vi "uTTA_Calibration_V2.vi"() -> ()   [LabVIEW 2021]
uses:
  <vilib>/Utility/miscctls.llb/LVPointTypeDef.ctl
  uTTA_Device_Driver/uTTA_Controls/CTL_uTTA_AnalogParameter.ctl
  uTTA_Device_Driver/uTTA_Controls/CTL_uTTA_OperatingMode.ctl
panel:
  in  "Tab Control":enum32{"Setup", "Calibration"}(tab)
  in  "Embedd Steps":bool caption="Embedd Calibration Steps in Main Window"
  in  "ADC Stage":bool=TRUE
  in  "Heating Current":bool=TRUE
  in  "Differential Amp":bool=TRUE
  in  "I_Sense":bool=TRUE
  in  "VISA DMM":refnum<visa-resource-name>="COM9"
  in  "Storage_Path":path=path "C:/temp/Eigenentwicklungen/GitHub/uTTA/060_Example_Measurement_Data/Calibration"
  in  "VISA Function Gen":refnum<visa-resource-name>="TCPIP0::192.168.1.54::inst0::INSTR"
  in  "uTTA COM":refnum<visa-resource-name>="COM35"
  in  "Start":bool
  out "PGA":i32
  out "Measurement Active":bool
  out "Queue":i32
  out "Communication Error":errorcluster
  out "RunTime Error":errorcluster
  out "Last Message":string
  out "Status":string="Exit"
  in  "stop":bool
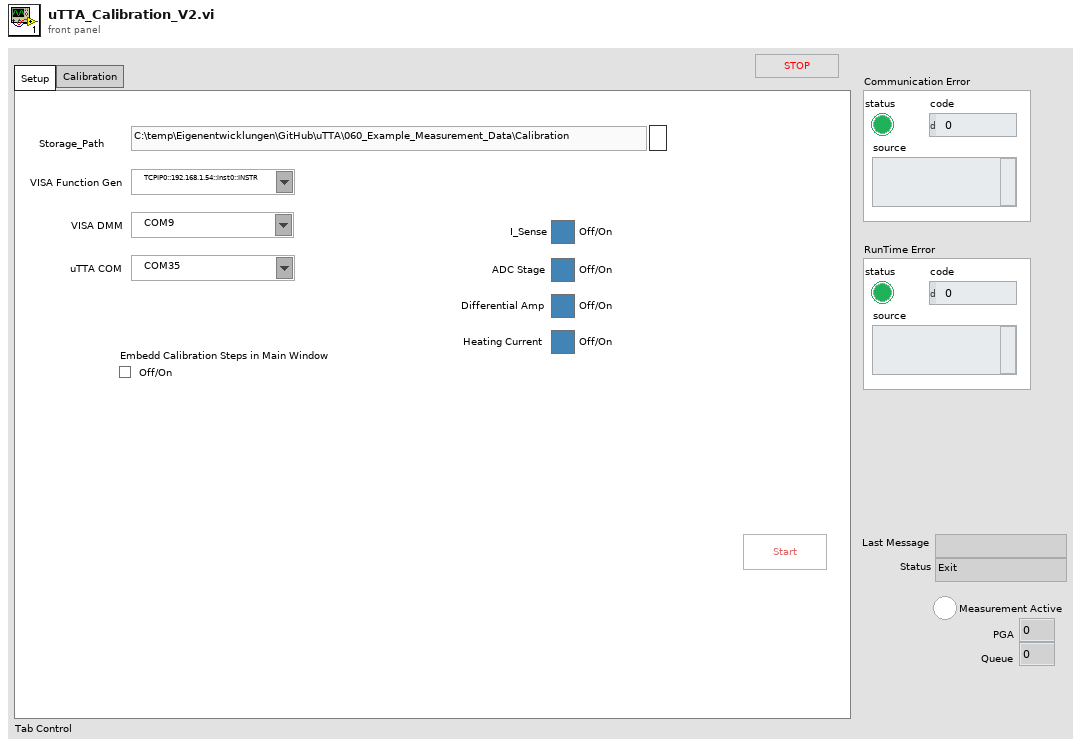
[diagram p1: front panel]
types:
  T1 = typedef "LVPointTypeDef.ctl" = cluster{"Horizontal":i16, "Vertical":i16}
  T2 = cluster{"ADC Values":i16[][], "Temperatures":dbl[][]}
  T3 = enum8{"Enabled", "Disabled", "Disabled and Grayed Out"}
  T4 = enum16{"open", "open or create", "create or replace", "create", "open (read-only)"}
  T5 = typedef "CTL_uTTA_AnalogParameter.ctl" = enum16{"ISEN", "SPARE", "VOFF"}
  T6 = typedef "CTL_uTTA_OperatingMode.ctl" = enum16{"NORMAL", "TEST_MODE", "TEMP_CONTROL"}
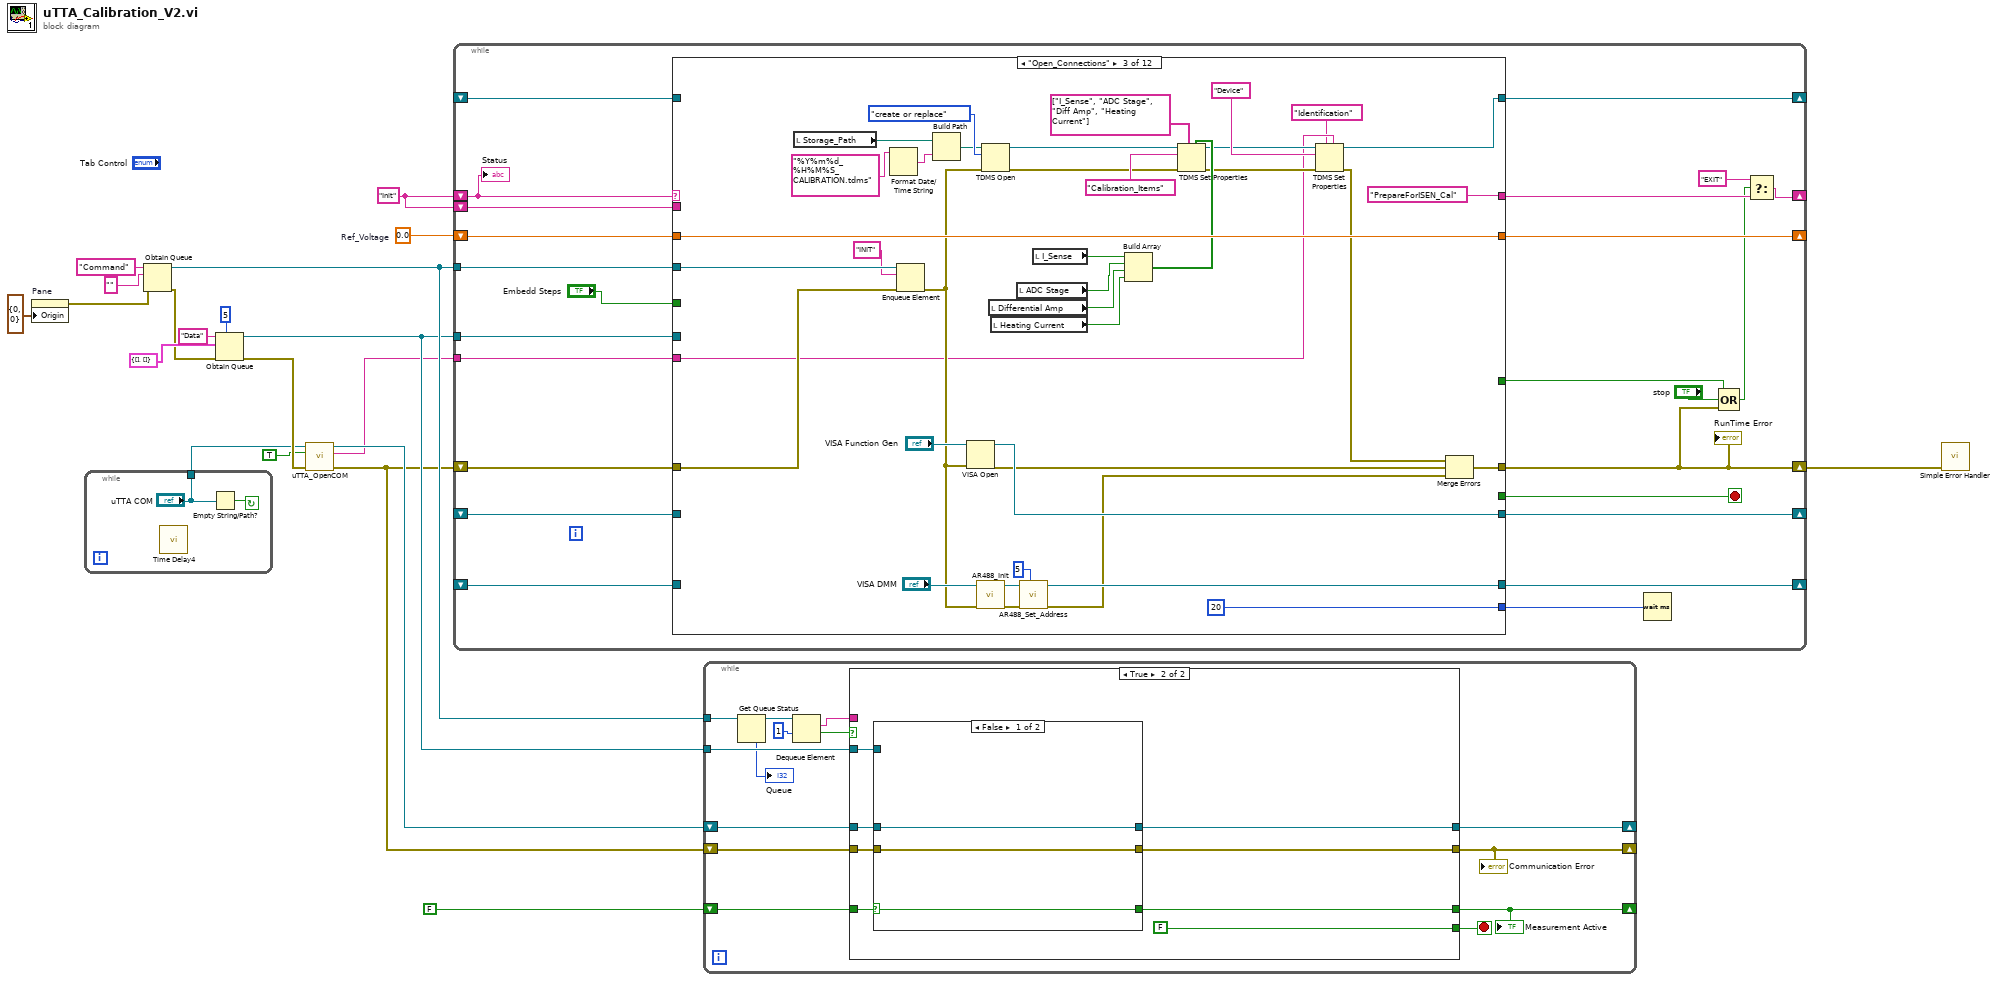
[diagram p0: block diagram]
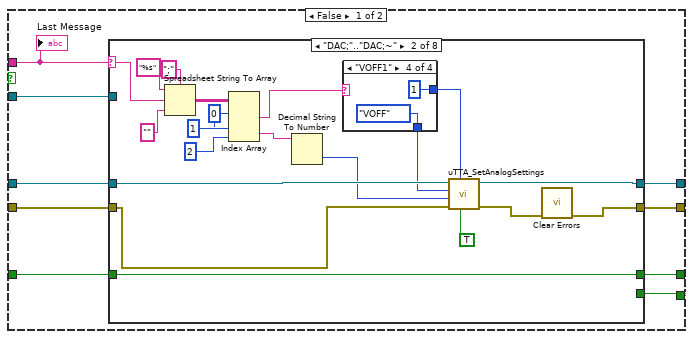
[diagram p2: hidden frame]
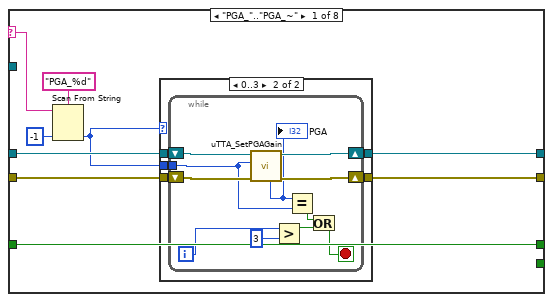
[diagram p3: hidden frame]
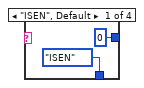
[diagram p5: hidden frame]
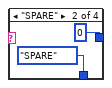
[diagram p6: hidden frame]
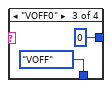
[diagram p7: hidden frame]
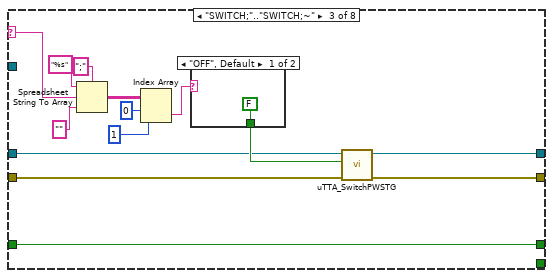
[diagram p8: hidden frame]
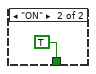
[diagram p9: hidden frame]
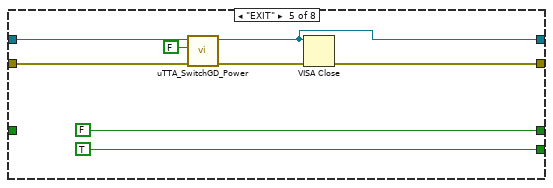
[diagram p11: hidden frame]
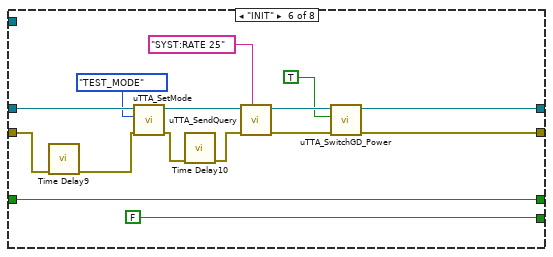
[diagram p12: hidden frame]
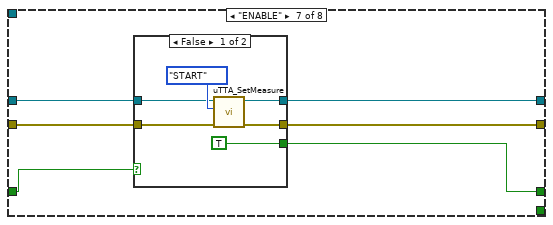
[diagram p13: hidden frame]
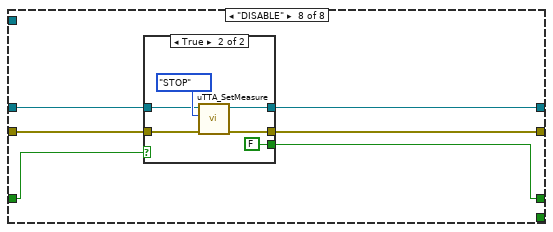
[diagram p15: hidden frame]
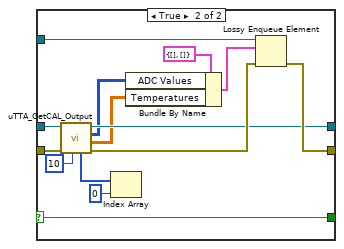
[diagram p17: hidden frame]
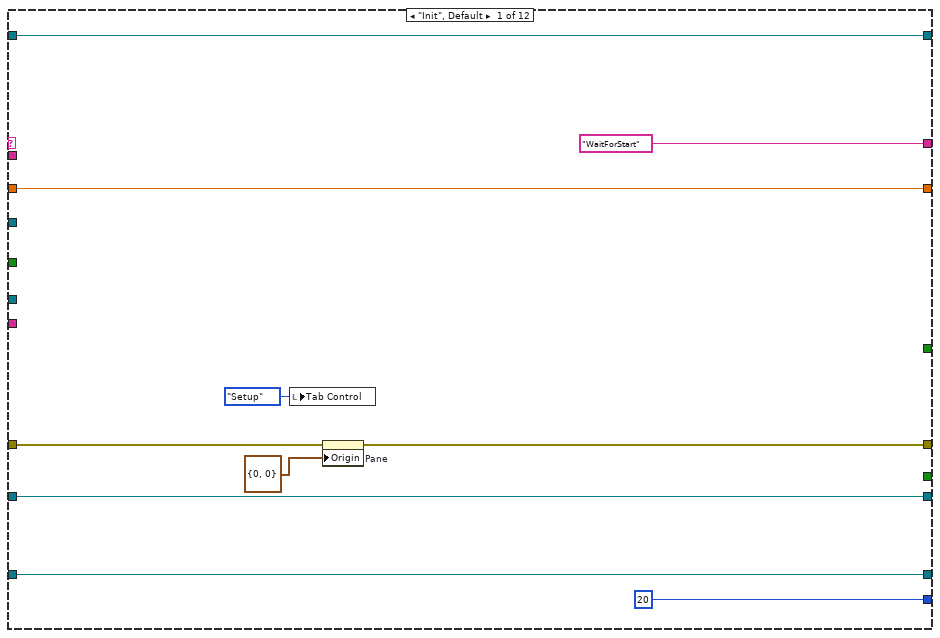
[diagram p18: hidden frame]
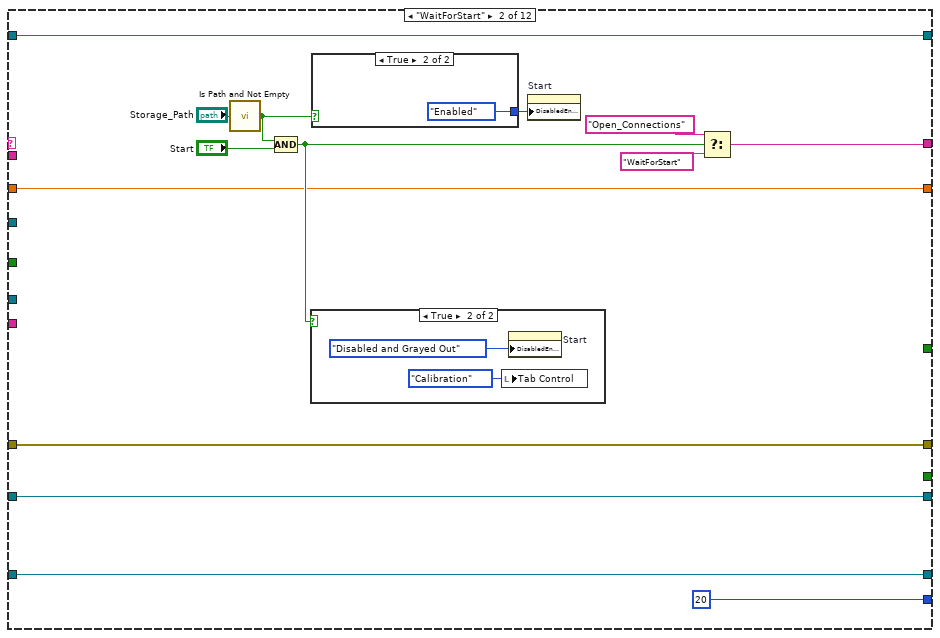
[diagram p19: hidden frame]
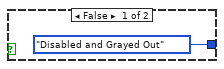
[diagram p20: hidden frame]
diagram:
  w11 = 0.0  # Ref_Voltage
  w10 = "Init"
  n1 = property on="Pane" class="Pane"("Origin"=T1 {"Horizontal"=0, "Vertical"=0}) -> (error out=w4:errorcluster)  [unwired: 2 in, 1 out]
  n2 = while {
    tunnel: ["uTTA COM"] -> w3
    stop <- w22 continue-if-true
    n3 = call "Time Delay4"() -> ()  [unwired: 11 in, 1 out]
    n4 = Empty String/Path?(string/path="uTTA COM") -> (empty?=w22:bool)
  }
  n5 = Obtain Queue(name (unnamed)="Command", element data type="" ("name (unnamed)"), error in (no error)=w4) -> (queue out=w14:refnum<queue>, error out=w15:errorcluster)  [unwired: 2 in, 1 out]
  n6 = Obtain Queue(max queue size (-1, unlimited)=5, name (unnamed)="Data", element data type=T2 {"ADC Values"=[], "Temperatures"=[]}, error in (no error)=w15) -> (queue out=w7:refnum<queue>, error out=w9:errorcluster)  [unwired: 1 in, 1 out]
  n7 = call "uTTA_OpenCOM.vi"("error in"=w9, "Log Serial Monitor(T)"=TRUE ("Log Serial Monitor"), "VISA in"=w3) -> ("error out"=w6:errorcluster, "Identity"=w1:string, "VISA out"=w8:refnum<visa-resource-name>)  [unwired: 6 in]
  n8 = while {
    shift-right: [w33] -> _
    shift-left: w10 -> [w44]
    shift-right: [w31] -> w13
    shift-left: w6 -> [w46]
    shift-right: [w42] -> _
    shift-left: _ -> [w43]
    shift-right: [w41] -> _
    shift-left: _ -> [w40]
    shift-left: w10 -> [w39]
    tunnel: w14 -> [w38]
    tunnel: w7 -> [w37]
    shift-right: [w35] -> _
    shift-left: w11 -> [w36]
    shift-right: [w27] -> _
    shift-left: _ -> [w26]
    tunnel: w1 -> [w23]
    stop <- w28 stop-if-true
    n9 = case shown="\"Open_Connections\"" w44 {
      selector: w44 -> [_ _ _ _ _ _ _ _ _ _ _ w261]
      tunnel: [_ _ _ _ _ _ _ _ _ _ _ TRUE] -> w28
      tunnel: w46 -> [w53 w70 w106 w117 w125 w151 w157 w184 w190 w220 w222 w244]
      tunnel: ["WaitForStart" ("t") w63 "PrepareForISEN_Cal" ("t") w114 "PrepareForADC_Cal" ("t") w147 "PrepareForDiffAmp_Cal" ("t") w180 "Prepare_for_Current_Cal" ("t") w214 "Exit" ("t") w261] -> w34
      tunnel: [w49 w70 w111 w117 w126 w151 w159 w184 w192 w220 w223 w252] -> w31
      tunnel: [u32 20 u32 20 u32 20 u32 20 u32 20 u32 20 u32 20 u32 20 u32 20 u32 10 u32 20 u32 10] -> w45
      tunnel: w43 -> [w52 w62 _ w120 w135 w150 w164 w183 w197 w219 w228 w243]
      tunnel: [w52 w62 w93 w120 w135 w150 w163 w183 w196 w219 w229 w243] -> w42
      tunnel: [w51 w61 w94 w118 w129 w149 w162 w182 w195 w218 w226 w254] -> w41
      tunnel: w40 -> [w51 w61 _ w118 w130 w149 w161 w182 w194 w218 w227 w254]
      tunnel: w39 -> [_ _ _ _ _ _ _ _ _ _ _ _]
      tunnel: w38 -> [_ _ w110 _ w132 _ w168 _ w201 _ w231 w246]
      tunnel: w37 -> [_ _ _ _ w131 _ w165 _ w198 _ w230 _]
      tunnel: w36 -> [w50 w60 w108 w121 w137 w153 w170 w186 w203 w217 w236 w258]
      tunnel: [w50 w60 w108 w121 w137 w153 w170 w186 w203 w217 w236 w258] -> w35
      tunnel: [w48 w58 w79 w119 w134 w152 w166 w185 w199 w216 w233 w251] -> w27
      tunnel: w26 -> [w48 w58 _ w119 w133 w152 w167 w185 w200 w216 w232 w251]
      tunnel: [_ _ _ _ w124 _ w156 _ w189 _ _ _] -> w25
      tunnel: "Embedd Steps" -> [_ _ _ _ w123 _ w155 _ w188 _ w221 _]
      tunnel: w23 -> [_ _ w76 _ _ _ _ _ _ _ _ _]
      frame "Init", Default {
        n10 = local write "Tab Control"(enum32{"Setup", "Calibration"}."Setup" ("Tab Control")) -> ()
        n11 = property on="Pane" class="Pane"(error in=w53, "Origin"=T1 {"Horizontal"=0, "Vertical"=0}) -> (error out=w49:errorcluster)  [unwired: 1 in, 1 out]
      }
      frame "WaitForStart" {
        n12 = call <vilib>:"Is Path and Not Empty.vi"("path"="Storage_Path") -> ("Is Path and Not Empty?"=w57:bool)  [unwired: 4 in]
        n13 = Compound Arithmetic op=AND(w57, "Start") -> (w64:bool)
        n14 = case shown="True" w64 {
          frame False {
          }
          frame True {
            n15 = local write "Tab Control"(enum32{"Setup", "Calibration"}."Calibration" ("Tab Control")) -> ()
            n16 = property on="Start" class="Bool"("DisabledEnum"=T3."Disabled and Grayed Out" ("Disabled")) -> ()  [unwired: 2 in, 2 out]
          }
        }
        n17 = case shown="True" w57 {
          tunnel: [T3."Disabled and Grayed Out" ("Disabled") T3."Enabled" ("Disabled")] -> w66
          frame False {
          }
          frame True {
          }
        }
        n18 = property on="Start" class="Bool"("DisabledEnum"=w66) -> ()  [unwired: 2 in, 2 out]
        n19 = Select(t="Open_Connections", s=w64, f="WaitForStart" ("t")) -> (s? t:f=w63:string)
      }
      frame "Open_Connections" {
        n20 = local read "Storage_Path"() -> (w102:path)
        n21 = Format Date/Time String(time format string (%c)="%Y%m%d_%H%M%S_CALIBRATION.tdms") -> (date/time string=w103:string)  [unwired: 2 in]
        n22 = Enqueue Element(queue=w110, element="INIT", error in (no error)=w106) -> (error out=w97:errorcluster)  [unwired: 1 in, 2 out]
        n23 = Build Path(base path=w102, name or relative path=w103) -> (appended path=w101:path)
        n24 = VISA Open(error in (no error)=w97, VISA resource name="VISA Function Gen") -> (VISA resource name=w93:refnum<visa-resource-name>, error out=w92:errorcluster)  [unwired: 3 in]
        n25 = call "AR488_Init.vi"("error in (no error)"=w97, "VISA Refnum in"="VISA DMM") -> ("error out"=w95:errorcluster, "VISA Refnum out"=w96:refnum<visa-resource-name>)  [unwired: 8 in]
        n26 = TDMS Open(8:w97, 10:T4."create or replace" ("operation (0:open)"), 11:w101) -> (0:w82:errorcluster, 3:w90:refnum<k34>)  [unwired: 4 in]
        n27 = local read "Differential Amp"() -> (w87:bool)
        n28 = local read "Heating Current"() -> (w86:bool)
        n29 = local read "ADC Stage"() -> (w88:bool)
        n30 = call "AR488_Set_Address.vi"("Address (0-31)"=u32 5, "error in"=w95, "VISA Refnum in"=w96) -> ("error out"=w91:errorcluster, "VISA Refnum out"=w94:refnum<visa-resource-name>)  [unwired: 7 in]
        n31 = local read "I_Sense"() -> (w89:bool)
        n32 = Build Array(w89, w88, w87, w86) -> (w83:bool[])
        n33 = TDMS Set Properties(5:w83, 7:string[] ["I_Sense", "ADC Stage", "Diff Amp", "Heating Current"], 8:w82, 10:"Calibration_Items" ("group name in (Untitled)"), 11:w90) -> (0:w77:errorcluster, 3:w80:refnum<k34>)  [unwired: 1 in, 2 out]
        n34 = TDMS Set Properties(5:w76, 7:"Identification", 8:w77, 10:"Device" ("group name in (Untitled)"), 11:w80) -> (0:w78:errorcluster, 3:w79:refnum<k34>)  [unwired: 1 in, 2 out]
        n35 = Merge Errors(w78, w92, w91) -> (w111:errorcluster)
      }
      frame "PrepareForISEN_Cal" {
        n36 = Select(t="ISEN_Cal", s="I_Sense", f="PrepareForADC_Cal" ("t")) -> (s? t:f=w114:string)
      }
      frame "ISEN_Cal" {
        n37 = case shown="False" w123 {
          tunnel: [w139 w144] -> w128
          tunnel: w125 -> [w139 w143]
          frame False {
          }
          frame True {
            n38 = Open VI Reference(vi path=path "C:/temp/Eigenentwicklungen/GitHub/uTTA/040_LabVIEW_GUI/uTTA/Calibration_Routine/SubVi/uTTA_Calibration_ISense.vi", error in (no error)=w143) -> (vi reference=w141:refnum<vi>, error out=w142:errorcluster)  [unwired: 4 in]
            n39 = invoke on="Sub Panel" class="SubPnl" method="Insert VI"(error in=w142, "VI Ref"=w141) -> (error out=w144:errorcluster)  [unwired: 2 in, 3 out]
          }
        }
        n40 = call "uTTA_Calibration_ISense.vi"("CommandQueue"=w132, "error in"=w128, "AR488_in"=w130, "DataQueue"=w131, "TDMS_FileIn"=w133) -> ("error out"=w127:errorcluster, "AR488_out"=w129:refnum<visa-resource-name>, "Abort"=w124:bool, "TDMS_FileOut"=w134:refnum<k34>)  [unwired: 1 in]
        n41 = invoke on="Sub Panel" class="SubPnl" method="Remove VI"(error in=w127) -> (error out=w126:errorcluster)  [unwired: 2 in, 2 out]
      }
      frame "PrepareForADC_Cal" {
        n42 = Select(t="ADC_Cal", s="ADC Stage", f="PrepareForDiffAmp_Cal") -> (s? t:f=w147:string)
      }
      frame "ADC_Cal" {
        n43 = case shown="False" w155 {
          tunnel: [w172 w177] -> w158
          tunnel: w157 -> [w172 w176]
          frame False {
          }
          frame True {
            n44 = Open VI Reference(vi path=path "C:/temp/Eigenentwicklungen/GitHub/uTTA/040_LabVIEW_GUI/uTTA/Calibration_Routine/SubVi/uTTA_Calibration_ADC.vi", error in (no error)=w176) -> (vi reference=w174:refnum<vi>, error out=w173:errorcluster)  [unwired: 4 in]
            n45 = invoke on="Sub Panel" class="SubPnl" method="Insert VI"(error in=w173, "VI Ref"=w174) -> (error out=w177:errorcluster)  [unwired: 2 in, 3 out]
          }
        }
        n46 = call "uTTA_Calibration_ADC.vi"("AR488_in"=w161, "CommandQueue"=w168, "error in"=w158, "FunctionGen_In"=w164, "DataQueue"=w165, "TDMS_FileIn"=w167) -> ("error out"=w160:errorcluster, "FunctionGen_Out"=w163:refnum<visa-resource-name>, "abort"=w156:bool, "TDMS_FileOut"=w166:refnum<k34>, "AR488_out"=w162:refnum<visa-resource-name>)  [unwired: 1 in]
        n47 = invoke on="Sub Panel" class="SubPnl" method="Remove VI"(error in=w160) -> (error out=w159:errorcluster)  [unwired: 2 in, 2 out]
      }
      frame "PrepareForDiffAmp_Cal" {
        n48 = Select(t="DiffAmp_Cal", s="Differential Amp", f="Prepare_for_Current_Cal") -> (s? t:f=w180:string)
      }
      frame "DiffAmp_Cal" {
        n49 = case shown="False" w188 {
          tunnel: [w205 w210] -> w191
          tunnel: w190 -> [w205 w206]
          frame False {
          }
          frame True {
            n50 = Open VI Reference(vi path=path "C:/temp/Eigenentwicklungen/GitHub/uTTA/040_LabVIEW_GUI/uTTA/Calibration_Routine/SubVi/uTTA_Calibration_DiffAmp.vi", error in (no error)=w206) -> (vi reference=w208:refnum<vi>, error out=w207:errorcluster)  [unwired: 4 in]
            n51 = invoke on="Sub Panel" class="SubPnl" method="Insert VI"(error in=w207, "VI Ref"=w208) -> (error out=w210:errorcluster)  [unwired: 2 in, 3 out]
          }
        }
        n52 = call "uTTA_Calibration_DiffAmp.vi"("AR488_in"=w194, "CommandQueue"=w201, "error in"=w191, "FunctionGen_In"=w197, "DataQueue"=w198, "TDMS_FileIn"=w200) -> ("error out"=w193:errorcluster, "FunctionGen_Out"=w196:refnum<visa-resource-name>, "aborted"=w189:bool, "TDMS_FileOut"=w199:refnum<k34>, "AR488_out"=w195:refnum<visa-resource-name>)  [unwired: 1 in]
        n53 = invoke on="Sub Panel" class="SubPnl" method="Remove VI"(error in=w193) -> (error out=w192:errorcluster)  [unwired: 2 in, 2 out]
      }
      frame "Prepare_for_Current_Cal" {
        n54 = Select(t="Current_Cal", s="Heating Current", f="Exit") -> (s? t:f=w214:string)
      }
      frame "Current_Cal" {
        n55 = case shown="False" w221 {
          tunnel: [w237 w242] -> w225
          tunnel: w222 -> [w237 w238]
          frame False {
          }
          frame True {
            n56 = Open VI Reference(vi path=path "C:/temp/Eigenentwicklungen/GitHub/uTTA/040_LabVIEW_GUI/uTTA/Calibration_Routine/SubVi/uTTA_Calibration_Curr.vi", error in (no error)=w238) -> (vi reference=w239:refnum<vi>, error out=w240:errorcluster)  [unwired: 4 in]
            n57 = invoke on="Sub Panel" class="SubPnl" method="Insert VI"(error in=w240, "VI Ref"=w239) -> (error out=w242:errorcluster)  [unwired: 2 in, 3 out]
          }
        }
        n58 = call "uTTA_Calibration_Curr.vi"("AR488_In"=w227, "CommandQueue"=w231, "error in"=w225, "FunctionGen_In"=w228, "DataQueue"=w230, "TDMS_FileIn"=w232) -> ("error out"=w224:errorcluster, "FunctionGen_Out"=w229:refnum<visa-resource-name>, "TDMS_FileOut"=w233:refnum<k34>, "AR488_Out"=w226:refnum<visa-resource-name>)  [unwired: 2 in]
        n59 = invoke on="Sub Panel" class="SubPnl" method="Remove VI"(error in=w224) -> (error out=w223:errorcluster)  [unwired: 2 in, 2 out]
      }
      frame "Exit" {
        n60 = Enqueue Element(queue=w246, element="DISABLE") -> (queue out=w247:refnum<queue>)  [unwired: 2 in, 2 out]
        n61 = TDMS Close(8:w244, 11:w251) -> (0:w249:errorcluster)  [unwired: 1 out]
        n62 = Flush Queue(queue=w247, error in (no error)=w249) -> (queue out=w250:refnum<queue>, error out=w248:errorcluster)  [unwired: 1 out]
        n63 = call "Time Delay3"("error in (no error)"=w248) -> ("error out"=w256:errorcluster)  [unwired: 10 in]
        n64 = Enqueue Element(queue=w250, element="EXIT", error in (no error)=w256) -> (error out=w253:errorcluster)  [unwired: 1 in, 2 out]
        n65 = VISA Close(VISA resource name=w243, error in (no error)=w253) -> (error out=w255:errorcluster)
        n66 = VISA Close(VISA resource name=w254, error in (no error)=w255) -> (error out=w252:errorcluster)
      }
    }
    "RunTime Error" <- w31
    n67 = Wait (ms)(milliseconds to wait=w45) -> ()  [unwired: 1 out]
    n68 = Compound Arithmetic op=OR(w25, "stop", w31) -> (w30:bool)
    n69 = Select(t="EXIT", s=w30, f=w34) -> (s? t:f=w33:string)
    "Status" <- w44
  }
  n70 = while {
    shift-right: [w273] -> _
    shift-left: w8 -> [w275]
    shift-right: [w272] -> _
    shift-left: w6 -> [w274]
    tunnel: w14 -> [w269]
    tunnel: w7 -> [w270]
    shift-right: [w264] -> _
    shift-left: FALSE -> [w265]
    stop <- w271 stop-if-true
    n71 = Get Queue Status(queue=w269) -> (queue out=w263:refnum<queue>, # elements in queue=→"Queue":i32)  [unwired: 2 in, 6 out]
    n72 = Dequeue Element(queue=w263, timeout in ms (-1)=1) -> (element=w266:string, timed out?=w267:bool)  [unwired: 1 in, 2 out]
    n73 = case shown="True" w267 {
      tunnel: w275 -> [w284 w417]
      tunnel: w274 -> [w283 w416]
      tunnel: [w282 w414] -> w273
      tunnel: [w281 w413] -> w272
      tunnel: [w280 FALSE] -> w271
      tunnel: w270 -> [w279 w412]
      tunnel: w266 -> [w276 _]
      tunnel: w265 -> [w278 w418]
      tunnel: [w277 w415] -> w264
      frame False {
        n74 = case shown="\"DAC;\"..\"DAC;~\"" w276 {
          selector: w276 -> [w292 w328 w343 _ _ _ _ _]
          tunnel: w284 -> [w289 w330 w341 w358 w362 w379 w386 w402]
          tunnel: w283 -> [w288 w326 w340 w357 w360 w377 w385 w401]
          tunnel: [w287 w316 w351 w358 w363 w369 w383 w400] -> w282
          tunnel: [w286 w314 w352 w357 w364 w370 w384 w399] -> w281
          tunnel: [_ _ _ _ TRUE FALSE _ _] -> w280
          tunnel: w279 -> [_ _ _ _ _ _ _ _]
          tunnel: w278 -> [w293 w331 w353 w356 _ w380 w382 w398]
          tunnel: [w293 w331 w353 w356 FALSE w380 w387 w397] -> w277
          frame "PGA_".."PGA_~" {
            n75 = Scan From String(format string="PGA_%d", input string=w292, default 1=-1 ("default value 1")) -> (output 1=w285:i32)  [unwired: 2 in, 3 out]
            n76 = case shown="0..3" w285 {
              tunnel: w285 -> [_ w300]
              tunnel: w289 -> [w295 w299]
              tunnel: w288 -> [w294 w298]
              tunnel: [w295 w297] -> w287
              tunnel: [w294 w296] -> w286
              frame Default {
              }
              frame 0..3 {
                n77 = while {
                  tunnel: w300 -> [w307]
                  shift-right: [w309] -> w297
                  shift-left: w299 -> [w311]
                  shift-right: [w308] -> w296
                  shift-left: w298 -> [w310]
                  i -> [w303]
                  stop <- w306 stop-if-true
                  n78 = call "uTTA_SetPGAGain.vi"("error in"=w310, "PGA Gain"=w307, "VISA Refnum in"=w311) -> ("error out"=w308:errorcluster, "VISA Refnum out"=w309:refnum<visa-resource-name>, "Set PGA Gain"=w301:u32)  [unwired: 5 in, 1 out]
                  "PGA" <- w301
                  n79 = Greater?(x=w303, y=3) -> (0:w304:bool)
                  n80 = Equal?(x=w301, y=w307) -> (x = y?=w305:bool)
                  n81 = Or(x=w305, y=w304) -> (x .or. y?=w306:bool)
                }
              }
            }
          }
          frame "DAC;".."DAC;~" {
            w323 = 0 ("index (row)")
            n82 = Spreadsheet String To Array(delimiter (Tab)=";", format string="%s", spreadsheet string=w328, array type (2D Dbl)="" ("default value 1")) -> (array=w325:string[][])
            n83 = Index Array(array=w325, index (row) #1=w323, index (col) #1=1 ("disabled index (col)"), index (row) #2=w323, index (col) #2=2 ("disabled index (col)")) -> (element #1=w321:string, element #2=w320:string)
            n84 = Decimal String To Number(string=w320) -> (number=w319:i32)  [unwired: 2 in, 1 out]
            n85 = case shown="\"VOFF1\"" w321 {
              tunnel: [CTL_uTTA_AnalogParameter."ISEN" ("Parameter") CTL_uTTA_AnalogParameter."SPARE" ("Parameter") CTL_uTTA_AnalogParameter."VOFF" ("Parameter") CTL_uTTA_AnalogParameter."VOFF" ("Parameter")] -> w313
              tunnel: [u32 0 ("Number") u32 0 ("Number") u32 0 ("Number") u32 1 ("Number")] -> w312
              frame "ISEN", Default {
              }
              frame "SPARE" {
              }
              frame "VOFF0" {
              }
              frame "VOFF1" {
              }
            }
            n86 = call "uTTA_SetAnalogSettings.vi"("Calibration Mode"=TRUE, "Number"=w312, "error in"=w326, "Set Value"=w319, "Parameter"=w313, "VISA Refnum in"=w330) -> ("error out"=w315:errorcluster, "VISA Refnum out"=w316:refnum<visa-resource-name>)  [unwired: 1 in, 1 out]
            n87 = call <vilib>:"Clear Errors.vi"("error in (no error)"=w315) -> ("error out"=w314:errorcluster)  [unwired: 5 in, 1 out]
          }
          frame "SWITCH;".."SWITCH;~" {
            n88 = Spreadsheet String To Array(delimiter (Tab)=";", format string="%s", spreadsheet string=w343, array type (2D Dbl)="" ("default value 1")) -> (array=w348:string[][])
            n89 = Index Array(array=w348, index (row)=0, index (col)=1 ("disabled index (col)")) -> (element=w345:string)
            n90 = case shown="\"OFF\", Default" w345 {
              tunnel: [FALSE ("Powerstage Enable") TRUE ("Powerstage Enable")] -> w342
              frame "OFF", Default {
              }
              frame "ON" {
              }
            }
            n91 = call "uTTA_SwitchPWSTG.vi"("error in"=w340, "Powerstage Enable"=w342, "VISA Refnum in"=w341) -> ("error out"=w352:errorcluster, "VISA Refnum out"=w351:refnum<visa-resource-name>)  [unwired: 2 in, 1 out]
          }
          frame Default {
          }
          frame "EXIT" {
            n92 = call "uTTA_SwitchGD_Power.vi"("error in"=w360, "GD Power Enable"=FALSE, "VISA Refnum in"=w362) -> ("error out"=w361:errorcluster, "VISA Refnum out"=w363:refnum<visa-resource-name>)  [unwired: 2 in, 1 out]
            n93 = VISA Close(VISA resource name=w363, error in (no error)=w361) -> (error out=w364:errorcluster)
          }
          frame "INIT" {
            n94 = call "Time Delay9"("error in (no error)"=w377) -> ("error out"=w376:errorcluster)  [unwired: 10 in]
            n95 = call "uTTA_SetMode.vi"("error in"=w376, "OperatingMode"=CTL_uTTA_OperatingMode."TEST_MODE", "VISA Refnum in"=w379) -> ("error out"=w375:errorcluster, "VISA Refnum out"=w378:refnum<visa-resource-name>)  [unwired: 2 in, 1 out]
            n96 = call "Time Delay10"("error in (no error)"=w375) -> ("error out"=w374:errorcluster)  [unwired: 10 in]
            n97 = call "uTTA_SendQuery.vi"("Send String"="SYST:RATE 25" ("write buffer"), "error in (no error)"=w374, "VISA Refnum in"=w378) -> ("error out"=w371:errorcluster, "VISA Refnum out"=w372:refnum<visa-resource-name>)  [unwired: 6 in, 1 out]
            n98 = call "uTTA_SwitchGD_Power.vi"("error in"=w371, "GD Power Enable"=TRUE, "VISA Refnum in"=w372) -> ("error out"=w370:errorcluster, "VISA Refnum out"=w369:refnum<visa-resource-name>)  [unwired: 2 in, 1 out]
          }
          frame "ENABLE" {
            n99 = case shown="False" w382 {
              selector: w382 -> [_ w394]
              tunnel: [TRUE w394] -> w387
              tunnel: w386 -> [w391 w396]
              tunnel: w385 -> [w390 w395]
              tunnel: [w389 w395] -> w384
              tunnel: [w388 w396] -> w383
              frame False {
                n100 = call "uTTA_SetMeasure.vi"("error in"=w390, "Action"=enum16{"STOP", "START"}."START", "VISA Refnum in"=w391) -> ("error out"=w389:errorcluster, "VISA Refnum out"=w388:refnum<visa-resource-name>)  [unwired: 2 in, 1 out]
              }
              frame True {
              }
            }
          }
          frame "DISABLE" {
            n101 = case shown="True" w398 {
              selector: w398 -> [w405 _]
              tunnel: w402 -> [w403 w410]
              tunnel: w401 -> [w404 w409]
              tunnel: [w403 w408] -> w400
              tunnel: [w404 w407] -> w399
              tunnel: [w405 FALSE] -> w397
              frame False {
              }
              frame True {
                n102 = call "uTTA_SetMeasure.vi"("error in"=w409, "Action"=enum16{"STOP", "START"}."STOP", "VISA Refnum in"=w410) -> ("error out"=w407:errorcluster, "VISA Refnum out"=w408:refnum<visa-resource-name>)  [unwired: 2 in, 1 out]
              }
            }
          }
        }
        "Last Message" <- w276
      }
      frame True {
        n103 = case shown="False" w418 {
          selector: w418 -> [w422 w436]
          tunnel: w417 -> [w421 w432]
          tunnel: w416 -> [w420 w431]
          tunnel: [w422 w436] -> w415
          tunnel: [w421 w429] -> w414
          tunnel: [w420 w433] -> w413
          tunnel: w412 -> [_ w435]
          frame False {
          }
          frame True {
            n104 = call "uTTA_GetCAL_Output.vi"("Number of Samples"=u32 10, "error in"=w431, "VISA Refnum in"=w432) -> ("error out"=w430:errorcluster, "Temperatures"=w427:dbl[][], "ADCs"=w428:i32[][], "VISA Refnum out"=w429:refnum<visa-resource-name>, "PGA"=w424:i32[])  [unwired: 4 in]
            n105 = Index Array(array=w424, index=0) -> ()  [unwired: 1 out]
            n106 = Bundle By Name(cluster=T2 {"ADC Values"=[], "Temperatures"=[]}, "ADC Values"=w428, "Temperatures"=w427) -> (w434:T2)
            n107 = Lossy Enqueue Element(queue=w435, element=w434, error in (no error)=w430) -> (error out=w433:errorcluster)  [unwired: 3 out]
          }
        }
      }
    }
    "Communication Error" <- w272
    "Measurement Active" <- w264
  }
  n108 = call <vilib>:"Simple Error Handler.vi"("error in (no error)"=w13) -> ()  [unwired: 4 in, 5 out]
